vi "clone.vi"(8 "error in (no error)":errorcluster, 11 "pRectangle in":refnum<class "pRectangle.lvclass">) -> (0 "error out":errorcluster, 3 "pRectangle out":refnum<class "pRectangle.lvclass">)   [LabVIEW 2018, in "pRectangle.lvclass"]
uses:
  pRectangle.lvclass
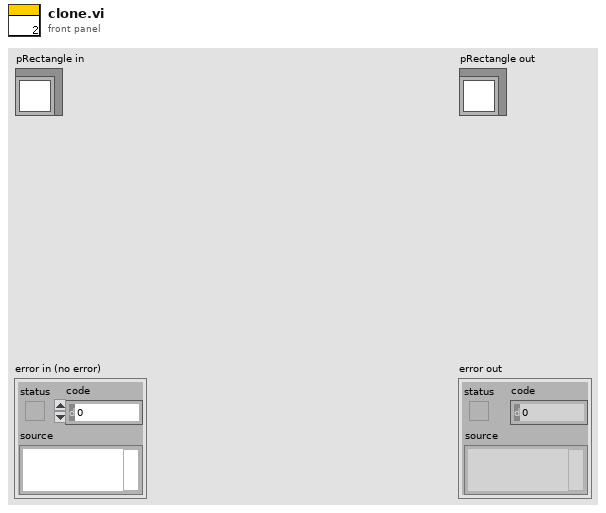
[diagram p1: front panel]
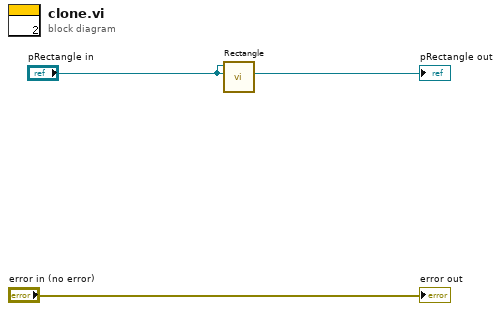
[diagram p0: block diagram]
diagram:
  n1 = call "Rectangle.vi"("target"="pRectangle in", "pRectangle in"="pRectangle in") -> ("pRectangle out"=→"pRectangle out":refnum<class "pRectangle.lvclass">)  [unwired: 8 in, 1 out]
  "error out" <- "error in (no error)"
